vi "16进制写入.vi"(1 "输入":string) -> (0 "输出":string)   [LabVIEW 2014]
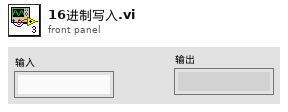
[diagram p1: front panel]
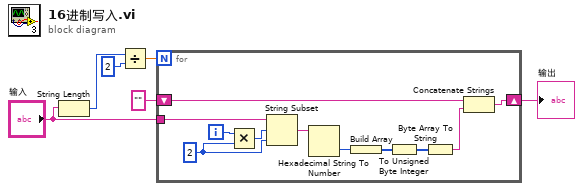
[diagram p0: block diagram]
diagram:
  n1 = String Length(string="输入") -> (length=w5:i32)
  n2 = Divide(x=w5, y=2 ("length")) -> (x/y=w3:dbl)
  n3 = for {
    N: w3 -> [_]
    tunnel: "输入" -> [w16]
    shift-right: [w12] -> w2
    shift-left: "" ("String") -> [w13]
    i -> [w11]
    w7 = 2 ("length (rest)")
    n4 = Multiply(x=w11, y=w7) -> (x*y=w10:i32)
    n5 = String Subset(string=w16, offset (0)=w10, length (rest)=w7) -> (substring=w15:string)
    n6 = Hexadecimal String To Number(string=w15) -> (number=w17:u32)  [unwired: 2 in, 1 out]
    n7 = Build Array(w17) -> (w9:u32[])
    n8 = To Unsigned Byte Integer(number=w9) -> (unsigned 8bit integer=w8:u8[])
    n9 = Byte Array To String(unsigned byte array=w8) -> (string=w14:string)
    n10 = Concatenate Strings(w13, w14) -> (w12:string)
  }
  "输出" <- w2
